vi "Move Camera.vi"(9 "Camera Speed":sgl=2.0, 10 "Camera Movement":T1, 11 "Scene in":refnum<class "Scene.lvclass">) -> (3 "Scene out":refnum<class "Scene.lvclass">)   [LabVIEW 2020, in "Scene.lvclass"]
uses:
  Scene.lvclass
  Scene.lvclass/Scene.ctl
  Graphics/Libraries/3D/3D.lvlib
  Graphics/Libraries/3D/Camera.ctl
  Camera Movement.ctl
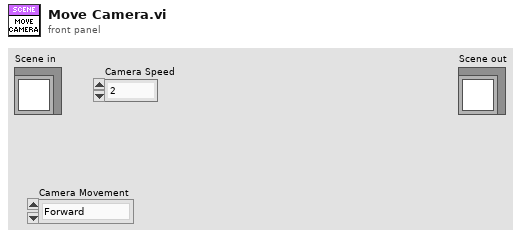
[diagram p1: front panel]
types:
  T1 = typedef "Scene.lvclass/Camera Movement.ctl" = enum16{"Forward", "Backwards", "Up", "Down", "Left", "Right", "Yaw CCW", "Yaw CW"}
  T2 = typedef "3D.lvlib/Camera.ctl" = cluster{"Field Of View":sgl, "Near Plane":sgl, "Far Plane":sgl}
  T3 = typedef "Raster.lvlib/Rectangle Dimensions.ctl" = cluster{"Width":u32, "Height":u32}
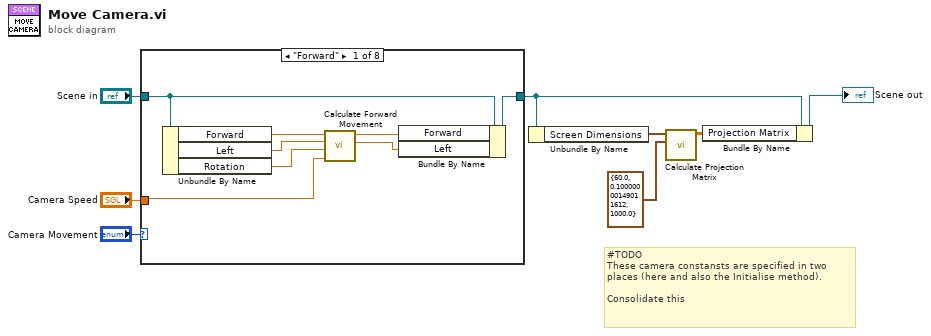
[diagram p0: block diagram]
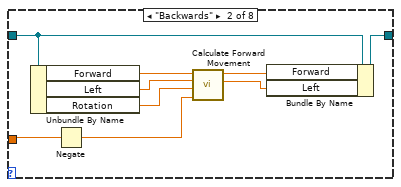
[diagram p2: hidden frame]
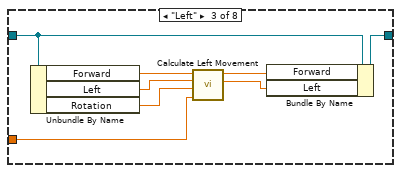
[diagram p3: hidden frame]
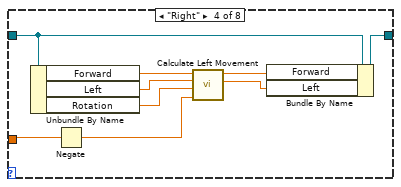
[diagram p4: hidden frame]
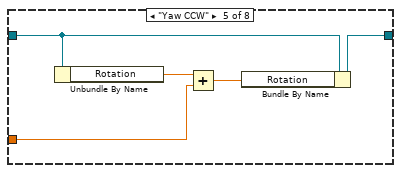
[diagram p5: hidden frame]
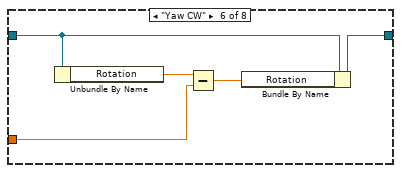
[diagram p6: hidden frame]
diagram:
  # "#TODO\nThese camera constansts are specified in two places (here and also the Initialise method).\n\nConsolidate this"
  n1 = case shown="\"Forward\"" "Camera Movement" {
    tunnel: "Scene in" -> [w16 w25 w33 w42 w47 w52 w53 w54]
    tunnel: "Camera Speed" -> [w11 w20 w28 w37 w46 w51 _ _]
    tunnel: [w13 w22 w30 w39 w43 w48 w53 w54] -> w6
    frame "Forward" {
      n2 = Unbundle By Name(w16) -> ("Forward"=w15:sgl, "Left"=w10:sgl, "Rotation"=w9:sgl)
      n3 = call "Calculate Forward Movement.vi"("Camera Speed"=w11, "Rotation"=w9, "Previous Left"=w10, "Previous Forward"=w15) -> ("Next Left"=w12:sgl, "Next Forward"=w14:sgl)  [unwired: 6 in]
      n4 = Bundle By Name(cluster=w16, "Forward"=w14, "Left"=w12) -> (w13:refnum<class "Scene.lvclass">)
    }
    frame "Backwards" {
      n5 = Unbundle By Name(w25) -> ("Forward"=w24:sgl, "Left"=w19:sgl, "Rotation"=w18:sgl)
      n6 = Negate(x=w20) -> (-x=w17:sgl)
      n7 = call "Calculate Forward Movement.vi"("Camera Speed"=w17, "Rotation"=w18, "Previous Left"=w19, "Previous Forward"=w24) -> ("Next Left"=w21:sgl, "Next Forward"=w23:sgl)  [unwired: 6 in]
      n8 = Bundle By Name(cluster=w25, "Forward"=w23, "Left"=w21) -> (w22:refnum<class "Scene.lvclass">)
    }
    frame "Left" {
      n9 = Unbundle By Name(w33) -> ("Forward"=w32:sgl, "Left"=w27:sgl, "Rotation"=w26:sgl)
      n10 = call "Calculate Left Movement.vi"("Camera Speed"=w28, "Rotation"=w26, "Previous Left"=w27, "Previous Forward"=w32) -> ("Next Left"=w29:sgl, "Next Forward"=w31:sgl)  [unwired: 6 in]
      n11 = Bundle By Name(cluster=w33, "Forward"=w31, "Left"=w29) -> (w30:refnum<class "Scene.lvclass">)
    }
    frame "Right" {
      n12 = Unbundle By Name(w42) -> ("Forward"=w41:sgl, "Left"=w36:sgl, "Rotation"=w35:sgl)
      n13 = Negate(x=w37) -> (-x=w34:sgl)
      n14 = call "Calculate Left Movement.vi"("Camera Speed"=w34, "Rotation"=w35, "Previous Left"=w36, "Previous Forward"=w41) -> ("Next Left"=w38:sgl, "Next Forward"=w40:sgl)  [unwired: 6 in]
      n15 = Bundle By Name(cluster=w42, "Forward"=w40, "Left"=w38) -> (w39:refnum<class "Scene.lvclass">)
    }
    frame "Yaw CCW" {
      n16 = Unbundle By Name(w47) -> ("Rotation"=w45:sgl)
      n17 = Add(x=w45, y=w46) -> (x+y=w44:sgl)
      n18 = Bundle By Name(cluster=w47, "Rotation"=w44) -> (w43:refnum<class "Scene.lvclass">)
    }
    frame "Yaw CW" {
      n19 = Unbundle By Name(w52) -> ("Rotation"=w50:sgl)
      n20 = Subtract(x=w50, y=w51) -> (x-y=w49:sgl)
      n21 = Bundle By Name(cluster=w52, "Rotation"=w49) -> (w48:refnum<class "Scene.lvclass">)
    }
    frame "Up" {
      # "#TODO"
    }
    frame "Down" {
      # "#TODO"
    }
  }
  n22 = Unbundle By Name(w6) -> ("Screen Dimensions"=w8:T3)
  n23 = call "Calculate Projection Matrix.vi"("Camera"=T2 {"Field Of View"=60.0, "Near Plane"=0.1, "Far Plane"=1000.0}, "Screen Dimensions"=w8) -> ("Projection Matrix"=w7:sgl[][])  [unwired: 9 in]
  n24 = Bundle By Name(cluster=w6, "Projection Matrix"=w7) -> (→"Scene out":refnum<class "Scene.lvclass">)
